vi "CfgManager.Text Test Launcher.vi"() -> ()   [LabVIEW 2013]
uses:
  source/Manager.Text/ConfigManager.Text.lvclass
  source/Manager/Decompose KVPs.vi
  source/Manager/Write.vi
  source/Manager/ConfigManager.lvclass
panel:
  out "Keys":string[](array[string])
  out "modified configuration":variant
  out "error out":errorcluster
  out "initial configuration":variant
  out "filepath":path
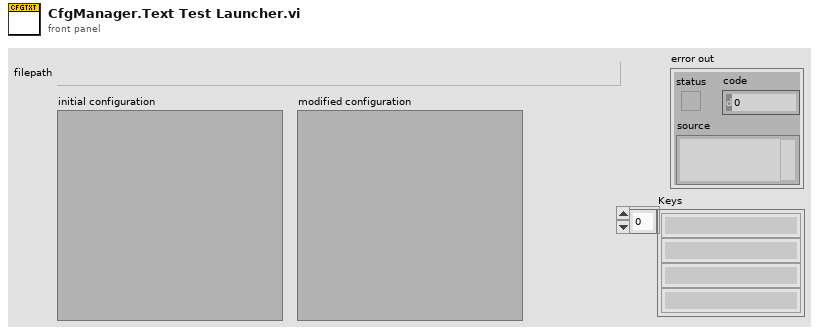
[diagram p1: front panel]
types:
  T1 = cluster{"String":string, "Numeric":dbl, "Boolean":bool}
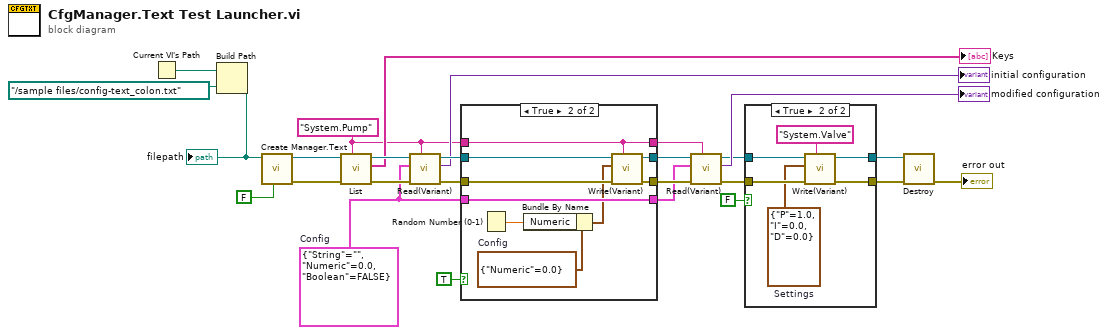
[diagram p0: block diagram]
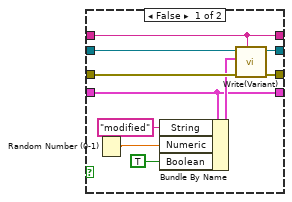
[diagram p2: hidden frame]
diagram:
  w9 = "System.Pump" ("Qualified Name")
  w6 = T1 {"String"="", "Numeric"=0.0, "Boolean"=FALSE}  # Config
  n1 = Current VI's Path() -> (path=w3:path)
  n2 = Build Path(base path=w3, name or relative path=path "../sample files/config-text_colon.txt" ("filepath 2")) -> (appended path=w1:path)
  "filepath" <- w1
  n3 = call "Create Manager.Text.vi"("read-only?"=FALSE, "filepath"=w1) -> ("error out"=w19:errorcluster, "ConfigManager.Text out"=w20:refnum<class "ConfigManager.Text.lvclass">)  [unwired: 7 in, 1 out]
  n4 = call "List.vi"("Qualified Name"=w9, "error in (no error)"=w19, "ConfigManager in"=w20) -> ("error out"=w18:errorcluster, "Keys"=→"Keys":string[], "ConfigManager out"=w17:refnum<class "ConfigManager.Text.lvclass">)  [unwired: 6 in]
  n5 = call "Read(Variant).vi"("Qualified Name"=w9, "error in (no error)"=w18, "Type"=w6, "ConfigManager in"=w17) -> ("error out"=w24:errorcluster, "value"=→"initial configuration":variant, "ConfigManager out"=w25:refnum<class "ConfigManager.Text.lvclass">)  [unwired: 3 in, 2 out]
  n6 = case shown="True" TRUE {
    tunnel: w25 -> [w33 w45]
    tunnel: w24 -> [w32 w44]
    tunnel: [w35 w43] -> w23
    tunnel: [w34 w42] -> w22
    tunnel: w9 -> [w36 w41]
    tunnel: [w36 w41] -> w7
    tunnel: w6 -> [w27 w40]
    tunnel: [w27 w40] -> w5
    frame False {
      n7 = Random Number (0-1)() -> (number: 0 to 1=w29:dbl)
      n8 = Bundle By Name(cluster=w27, "String"="modified", "Numeric"=w29, "Boolean"=TRUE) -> (w28:T1)
      n9 = call "Write(Variant).vi"("Qualified Name"=w36, "error in (no error)"=w32, "value"=w28, "ConfigManager in"=w33) -> ("error out"=w34:errorcluster, "ConfigManager out"=w35:refnum<class "ConfigManager.Text.lvclass">)  [unwired: 5 in, 1 out]
    }
    frame True {
      w39 = cluster{"Numeric":dbl} {"Numeric"=0.0}  # Config
      n10 = Random Number (0-1)() -> (number: 0 to 1=w38:dbl)
      n11 = Bundle By Name(cluster=w39, "Numeric"=w38) -> (w37:cluster{"Numeric":dbl})
      n12 = call "Write(Variant).vi"("Qualified Name"=w41, "error in (no error)"=w44, "value"=w37, "ConfigManager in"=w45) -> ("error out"=w42:errorcluster, "ConfigManager out"=w43:refnum<class "ConfigManager.Text.lvclass">)  [unwired: 5 in, 1 out]
    }
  }
  n13 = call "Read(Variant).vi"("Qualified Name"=w7, "error in (no error)"=w22, "Type"=w5, "ConfigManager in"=w23) -> ("error out"=w12:errorcluster, "value"=→"modified configuration":variant, "ConfigManager out"=w14:refnum<class "ConfigManager.Text.lvclass">)  [unwired: 3 in, 2 out]
  n14 = case shown="True" FALSE {
    tunnel: w14 -> [w47 w53]
    tunnel: [w47 w52] -> w13
    tunnel: w12 -> [w46 w51]
    tunnel: [w46 w50] -> w11
    frame False {
    }
    frame True {
      w48 = cluster{"P":dbl, "I":dbl, "D":dbl} {"P"=1.0, "I"=0.0, "D"=0.0}  # Settings
      n15 = call "Write(Variant).vi"("Qualified Name"="System.Valve", "error in (no error)"=w51, "value"=w48, "ConfigManager in"=w53) -> ("error out"=w50:errorcluster, "ConfigManager out"=w52:refnum<class "ConfigManager.Text.lvclass">)  [unwired: 5 in, 1 out]
    }
  }
  n16 = call-dynamic "Destroy.vi"("error in (no error)"=w11, "ConfigManager.Text in"=w13) -> ("error out"=→"error out":errorcluster)  [unwired: 8 in, 1 out]
